vi "CPP-AQ.vi"() -> (5 "Plug in titles":string[](array[string]), 7 "Plug in values":string[](array[string]))   [LabVIEW 2016]
uses:
  <vilib>/Utility/miscctls.llb/LVPositionTypeDef.ctl
  <vilib>/Utility/miscctls.llb/LVForegroundBackgroundColorsTypeDef.ctl
  Globals/Meas_global.vi
  CPPSW/CPP Global.vi
panel:
  in  "Tab Control":enum32{"FID Traces", "Numerics"}(tab)
  out "FID Means":T1(graph)
  out "FID PPM":cluster{"Time (s)":dbl[], "Eng Values":dbl[]}[](graph)
  out "COV(%)":dbl[](array[numeric])
  out "sigma(ppm)":dbl[](array[numeric])
  out "DeltaMean(ppm)":dbl[](array[numeric])
  in  "Blocks":i32
  out "FIDsymbol":string[](array[string])
  out "PPM":dbl[](array[numeric]) format="%.1f"
  # "Avg PPM Above BG"
  # "https://en.wikipedia.org/wiki/Coefficient_of_variation"
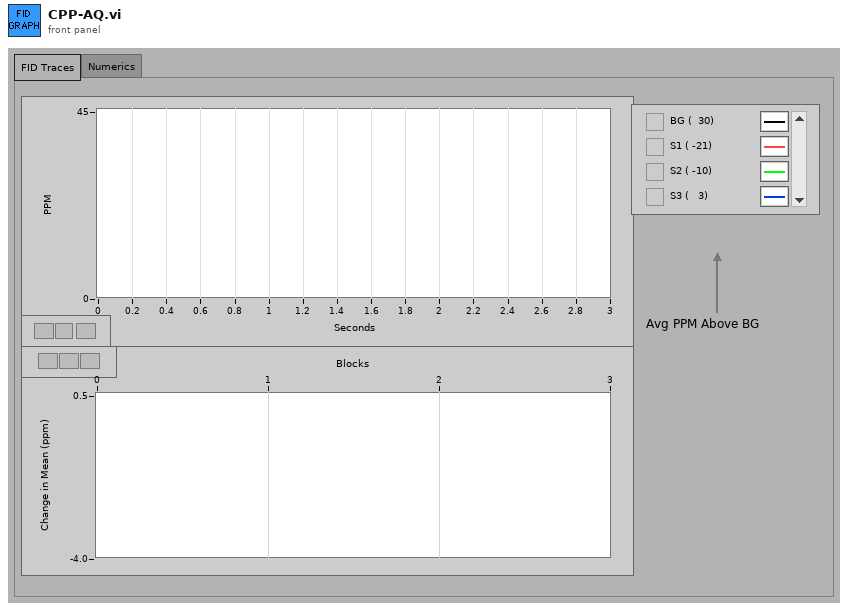
[diagram p1: front panel]
types:
  T1 = cluster{"[0]":dbl, "[1]":dbl, "[2]":dbl, "[3]":dbl}
  T2 = typedef "Analysis_info_cluster.ctl" = cluster{"Colour":u32, "Inst type":T3, "Inst name":string, "Symbol":string, "Code name":string, "Extra Info":string, "Inst Array":T4, "Extra Titles":string[], "Extra Values":string[], "U":dbl, "u^2":dbl, "u^3":dbl, "u^4":dbl, "Skew_u":dbl, "Kurt_u":dbl, "Sd Error in Mean":dbl, "% u'/U":dbl, "X":dbl, "Y":dbl, "Z":dbl, "Timescale integral Estimate":dbl, "Sd Error in Variance":dbl, "Calib File":path, "Calib Constants":dbl[], "Output Position":bool, "Full Stats":bool, "Av Sampling Rate":dbl, "Av No of Samples":dbl, "Total Meas Time (s)":dbl, "ADAM Ch Name":string, "Max value":dbl, "Min value":dbl}
  T3 = typedef "Inst_type.ctl" = enum16{"Propeller anemometer", "Raw voltage", "Pressure Transducer", "Pitot-static tube", "Preston tube", "Hot wire", "Cross wire 1", "Cross wire 2", "Generic Linear", "Generic Polynomial", "Generic BackPoly", "Fast FID", "Thermocouple", "Cold wire", "Pulsed Wire", "LDA Vel", "LDA Tran time", "LDA Arr time", "Microphone"}
  T4 = typedef "Instrument_Array.ctl" = enum16{"PWA", "LDA", "Analogue"}
  T5 = typedef "Time_Trace_Cluster.ctl" = cluster{"Weighting":dbl[], "Time (s)":dbl[], "Voltage":dbl[], "Eng Values":dbl[]}
  T6 = cluster{"[0]":dbl, "[1]":dbl, "[2]":dbl, "[3]":dbl}[]
  T7 = typedef "FIDmapping.ctl" = cluster{"Run #":dbl, "Run Suffix":u16, "Receptor #":u16, "ReceptorID":u16, "FIDname":string, "Long\nRun?":bool}[]
  T8 = cluster{"Receptor IDs":string[], "Receptor Numbers":u16[]}
  T9 = cluster{"Run #":dbl, "Run Suffix":u16, "Receptor #":u16, "ReceptorID":u16, "FIDname":string, "Long\nRun?":bool}
  T10 = typedef "LVPositionTypeDef.ctl" = cluster{"Left":i32, "Top":i32}
  T11 = typedef "LVForegroundBackgroundColorsTypeDef.ctl" = cluster{"Foreground Color":u32, "Background Color":u32}
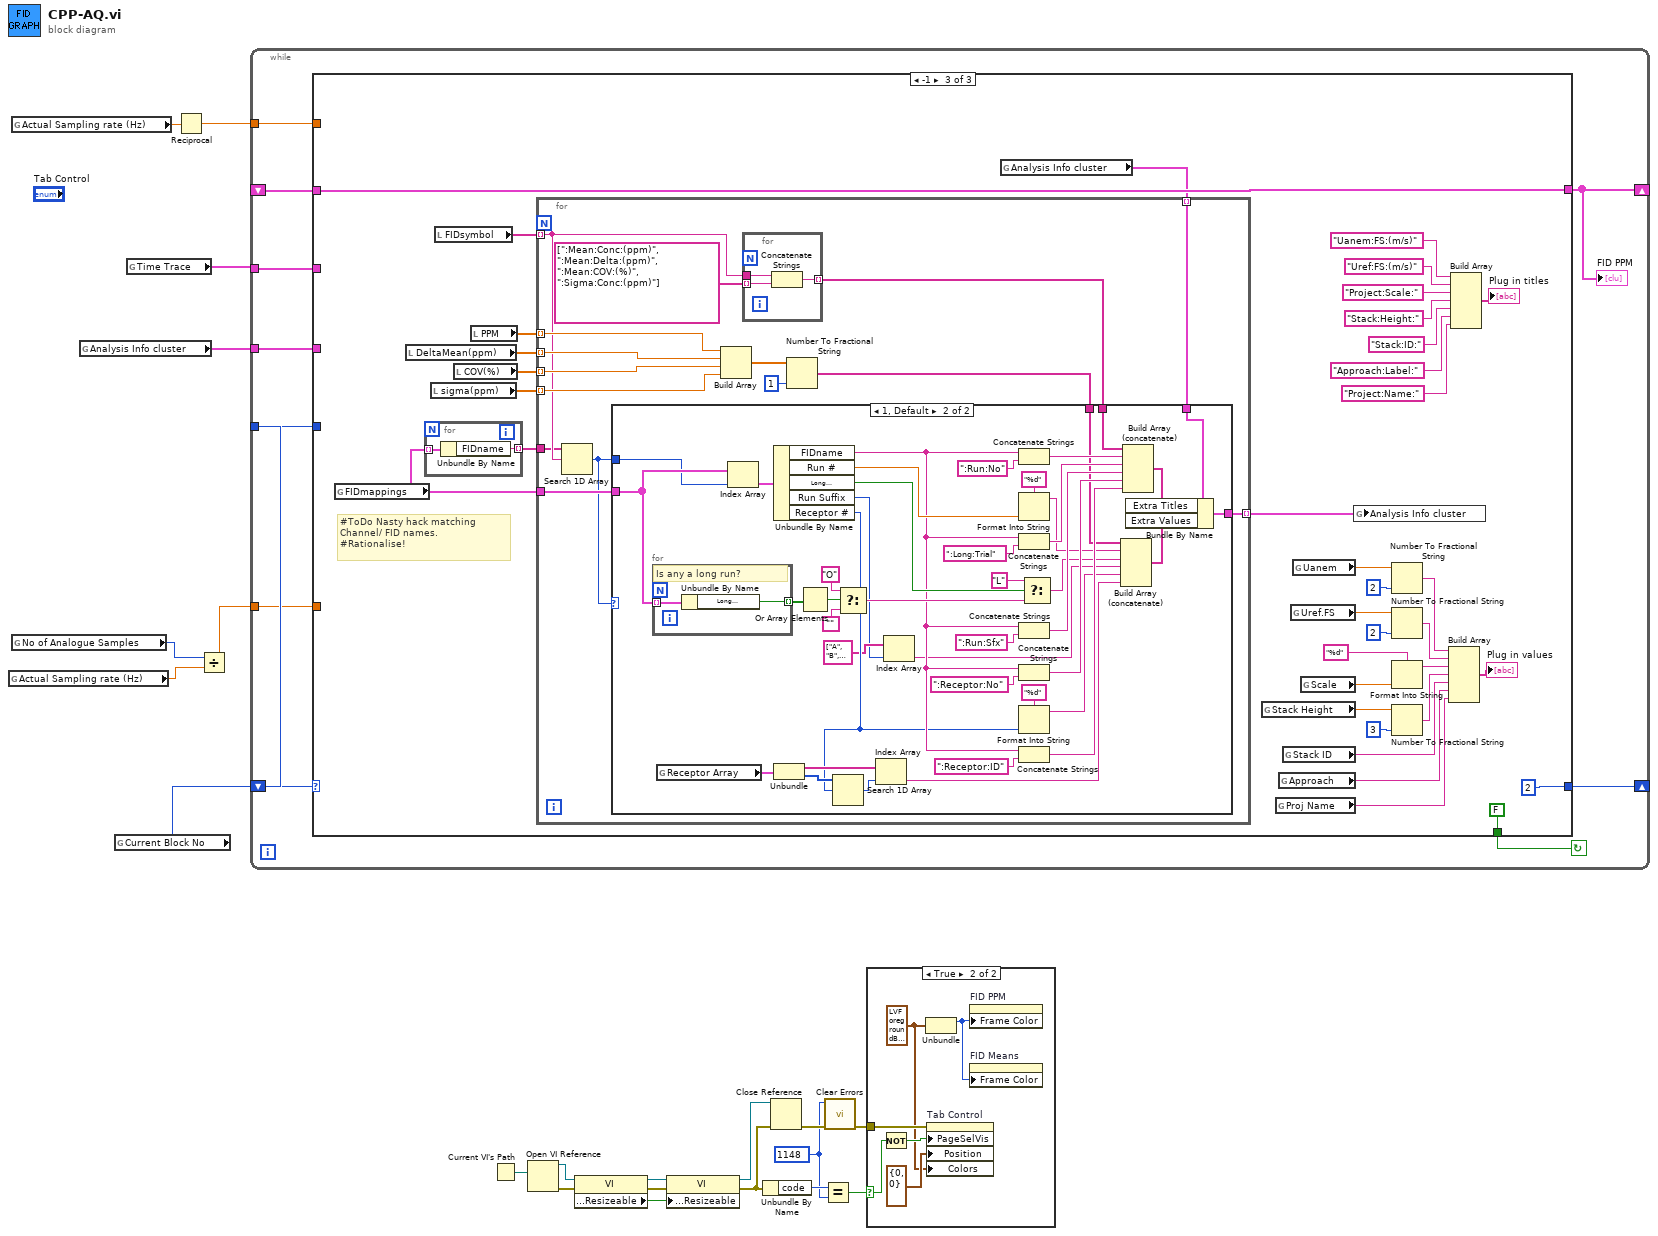
[diagram p0: block diagram]
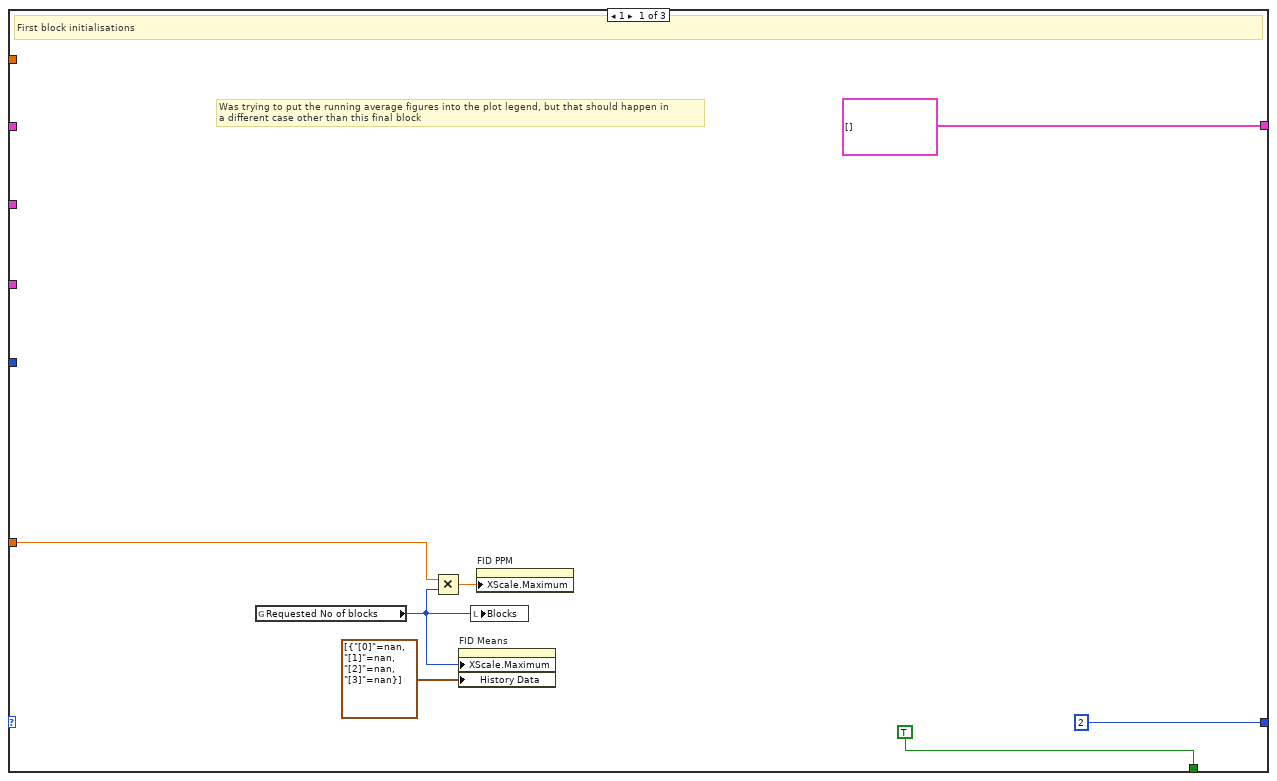
[diagram p3: hidden frame]
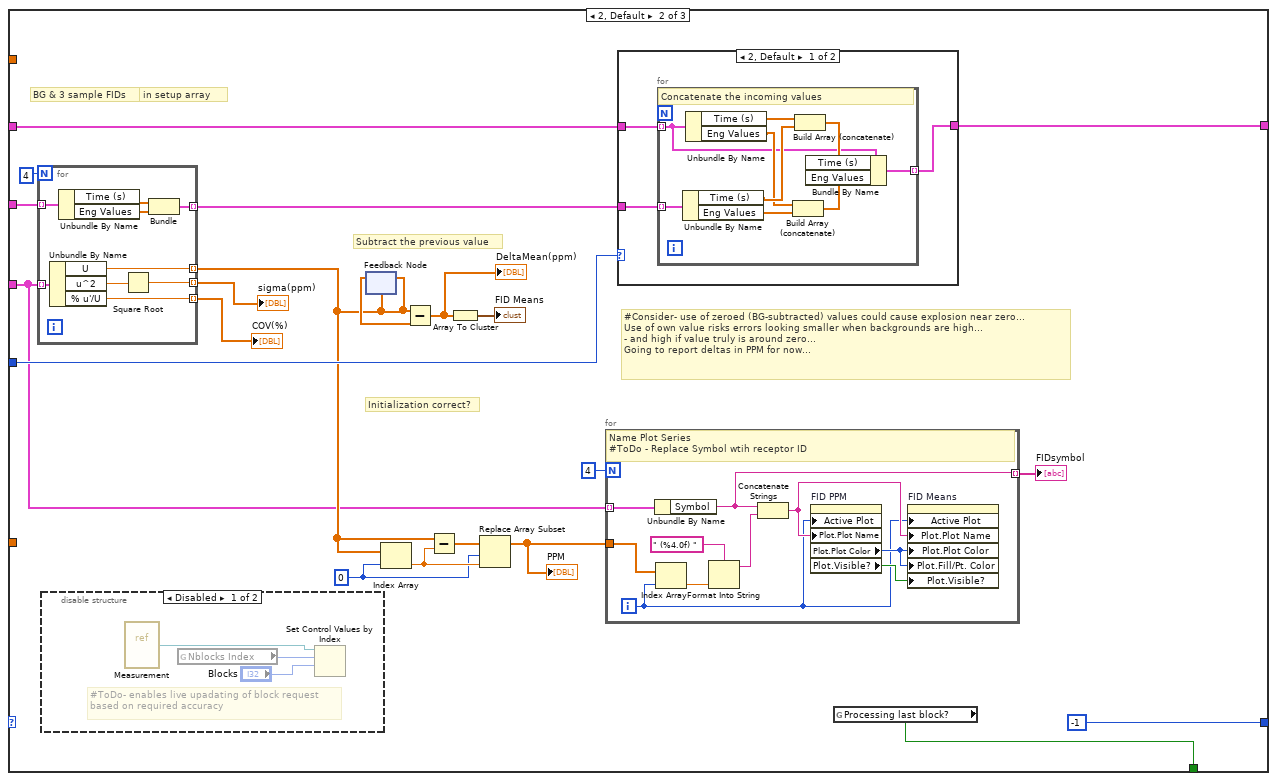
[diagram p4: hidden frame]
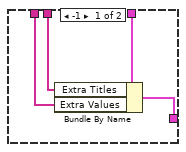
[diagram p7: hidden frame]
diagram:
  w3 = 1148 ("y")
  n1 = global read "Meas_global.vi" "Actual Sampling rate (Hz)"() -> (w17:dbl)
  n2 = global read "Meas_global.vi" "Actual Sampling rate (Hz)"() -> (w20:dbl)
  n3 = global read "Meas_global.vi" "No of Analogue Samples"() -> (w16:i32)
  n4 = global read "Meas_global.vi" "Analysis Info cluster"() -> (w14:T2[])
  n5 = global read "Meas_global.vi" "Current Block No"() -> (w18:i32)
  n6 = global read "Meas_global.vi" "Time Trace"() -> (w21:T5[])
  n7 = Reciprocal(x=w20) -> (1/x=w19:dbl)
  n8 = Divide(x=w16, y=w17) -> (x/y=w15:dbl)
  n9 = while {
    shift-left: w18 -> [w28]
    shift-right: [w29] -> _
    tunnel: w21 -> [w30]
    tunnel: w19 -> [w24]
    tunnel: w18 -> [w27]
    tunnel: w15 -> [w25]
    tunnel: w14 -> [w26]
    shift-right: [w22] -> _
    shift-left: _ -> [w23]
    stop <- w31 continue-if-true
    n10 = case shown="-1" w28 {
      tunnel: [TRUE w58 FALSE] -> w31
      tunnel: w30 -> [_ w59 _]
      tunnel: w24 -> [_ _ _]
      tunnel: [2 -1 ("Case") 2 ("Case")] -> w29
      tunnel: w27 -> [_ w51 _]
      tunnel: w25 -> [w35 _ _]
      tunnel: w26 -> [_ w39 _]
      tunnel: [cluster{"Time (s)":dbl[], "Eng Values":dbl[]}[] [] w52 w128] -> w22
      tunnel: w23 -> [_ w53 w128]
      frame 1 {
        # "Was trying to put the running average figures into the plot legend, but that should happen in\na different case other than this final block"
        # "First block initialisations"
        n11 = global read "Meas_global.vi" "Requested No of blocks"() -> (w32:i32)
        n12 = Multiply(x=w35, y=w32) -> (x*y=w36:dbl)
        n13 = property on="FID Means" class="WFChart (strict)"("XScale.Maximum"=w32, "History Data"=T6 [{"[0]"=nan, "[1]"=nan, "[2]"=nan, "[3]"=nan}]) -> ()  [unwired: 2 in, 2 out]
        n14 = local write "Blocks"(w32) -> ()
        n15 = property on="FID PPM" class="XYGraph (strict)"("XScale.Maximum"=w36) -> ()  [unwired: 2 in, 2 out]
      }
      frame 2, Default {
        w47 = 0 ("index")
        # "Initialization correct?"
        # "#Consider- use of zeroed (BG-subtracted) values could cause explosion near zero...\nUse of own value risks errors looking smaller when backgrounds are high...\n- and high if value truly is around zero...\nGoing to report deltas in PPM for now..."
        # "Subtract the previous value"
        # "BG FID is first element in setup array"
        # "BG & 3 sample FIDs"
        n16 = for {
          N: 4 -> [_]
          tunnel: w59 -> [w94] mode=indexing
          tunnel: w39 -> [w93] mode=indexing
          tunnel: [w92] -> w44 mode=indexing
          tunnel: [w89] -> w54 mode=indexing
          tunnel: [w87] -> w46 mode=indexing
          tunnel: [w86] -> w45 mode=indexing
          n17 = Unbundle By Name(w93) -> ("U"=w92:dbl, "u^2"=w88:dbl, "% u'/U"=w86:dbl)
          n18 = Unbundle By Name(w94) -> ("Time (s)"=w91:dbl[], "Eng Values"=w90:dbl[])
          n19 = Square Root(x=w88) -> (sqrt(x)=w87:dbl)
          n20 = Bundle("Time (s)"=w91, "Eng Values"=w90) -> (w89:cluster{"Time (s)":dbl[], "Eng Values":dbl[]})  [unwired: 1 in]
        }
        "sigma(ppm)" <- w46
        "COV(%)" <- w45
        n21 = disable-structure shown="Disabled" {
          frame Disabled {
            # "#ToDo- enables live upadating of block request based on required accuracy"
            n22 = vi-ref "Measurement.vi"() -> (w61:refnum<vi>)
            n23 = global read "Meas_global.vi" "Nblocks Index"() -> (w62:i32)
            n24 = Set Control Values by Index(0:w61, 1:w62, 2:"Blocks") -> ()  [unwired: 1 in, 1 out]
          }
          frame Enabled {
          }
        }
        n25 = feedback-in #1(w44) -> ()
        n26 = feedback #1(w44) -> (w55:dbl[])
        n27 = Index Array(array=w44, index=w47) -> (element=w48:dbl)
        n28 = Subtract(x=w44, y=w55) -> (x-y=w43:dbl[])
        "DeltaMean(ppm)" <- w43
        n29 = Subtract(x=w44, y=w48) -> (x-y=w49:dbl[])
        n30 = Array To Cluster(array=w43) -> (cluster=→"FID Means":T1)
        n31 = Replace Array Subset(array=w49, new element=w48, index=w47) -> (w40:dbl[])
        "PPM" <- w40
        n32 = for {
          N: 4 -> [_]
          tunnel: w39 -> [w72] mode=indexing
          tunnel: [w63] -> w41 mode=indexing
          tunnel: w40 -> [w66]
          i -> [w65]
          # "Name Plot Series\n#ToDo - Replace Symbol wtih receptor ID"
          n33 = Unbundle By Name(w72) -> ("Symbol"=w63:string)
          n34 = Index Array(array=w66, index=w65) -> (element=w64:dbl)
          n35 = Format Into String(format string=" (%4.0f) ", w64) -> (resulting string=w67:string)  [unwired: 2 in, 1 out]
          n36 = Concatenate Strings(w63, w67) -> (w69:string)
          n37 = property on="FID PPM" class="XYGraph (strict)"("Active Plot"=w65, "Plot.Plot Name"=w69) -> ("Plot.Plot Color"=w71:u32, "Plot.Visible?"=w70:bool)  [unwired: 2 in, 2 out]
          n38 = property on="FID Means" class="WFChart (strict)"("Active Plot"=w65, "Plot.Plot Name"=w69, "Plot.Plot Color"=w71, "Plot.Fill/Pt. Color"=w71, "Plot.Visible?"=w70) -> ()  [unwired: 2 in, 2 out]
        }
        "FIDsymbol" <- w41
        n39 = case shown="2, Default" w51 {
          tunnel: [w73 w85] -> w52
          tunnel: w54 -> [w75 w85]
          tunnel: w53 -> [w74 _]
          frame 2, Default {
            n40 = for {
              tunnel: w74 -> [w77] mode=indexing
              tunnel: w75 -> [w76] mode=indexing
              tunnel: [w78] -> w73 mode=indexing
              # "Concatenate the incoming values"
              n41 = Unbundle By Name(w76) -> ("Time (s)"=w83:dbl[], "Eng Values"=w82:dbl[])
              n42 = Unbundle By Name(w77) -> ("Time (s)"=w84:dbl[], "Eng Values"=w81:dbl[])
              n43 = Build Array (concatenate)(w81, w82) -> (w79:dbl[])
              n44 = Build Array (concatenate)(w84, w83) -> (w80:dbl[])
              n45 = Bundle By Name(cluster=w77, "Time (s)"=w80, "Eng Values"=w79) -> (w78:cluster{"Time (s)":dbl[], "Eng Values":dbl[]})
            }
          }
          frame 1 {
            # "Initialise with first block of data"
          }
        }
        n46 = global read "Meas_global.vi" "Processing last block?"() -> (w58:bool)
      }
      frame -1 {
        # "#ToDo Nasty hack matching Channel/ FID names.\n#Rationalise!"
        n47 = global read "CPP Global.vi" "FIDmappings"() -> (w120:T7)
        n48 = local read "DeltaMean(ppm)"() -> (w122:dbl[])
        n49 = for {
          tunnel: w120 -> [w132] mode=indexing
          tunnel: [w131] -> w119 mode=indexing
          n50 = Unbundle By Name(w132) -> ("FIDname"=w131:string)
        }
        n51 = local read "sigma(ppm)"() -> (w123:dbl[])
        n52 = local read "FIDsymbol"() -> (w127:string[])
        n53 = local read "COV(%)"() -> (w121:dbl[])
        n54 = local read "PPM"() -> (w124:dbl[])
        n55 = global read "Meas_global.vi" "Analysis Info cluster"() -> (w126:T2[])
        n56 = for {
          tunnel: w127 -> [w135] mode=indexing
          tunnel: w126 -> [w144] mode=indexing
          tunnel: [w143] -> w125 mode=indexing
          tunnel: w124 -> [w142] mode=indexing
          tunnel: w123 -> [w141] mode=indexing
          tunnel: w122 -> [w140] mode=indexing
          tunnel: w121 -> [w139] mode=indexing
          tunnel: w120 -> [w138]
          tunnel: w119 -> [w134]
          n57 = Search 1D Array(1D array=w134, element=w135) -> (index of element=w133:i32)  [unwired: 1 in]
          n58 = Build Array(w142, w140, w139, w141) -> (w147:dbl[])
          n59 = for {
            tunnel: w135 -> [w198]
            tunnel: string[] [":Mean:Conc:(ppm)", ":Mean:Delta:(ppm)", ":Mean:COV:(%)", ":Sigma:Conc:(ppm)"] -> [w197] mode=indexing
            tunnel: [w196] -> w137 mode=indexing
            n60 = Concatenate Strings(w198, w197) -> (w196:string)
          }
          n61 = Number To Fractional String(number=w147, precision (6)=i16 1) -> (F-format string=w136:string[])  [unwired: 2 in]
          n62 = case shown="1, Default" w133 {
            tunnel: w144 -> [w151 w193]
            tunnel: [w150 w192] -> w143
            tunnel: w138 -> [_ w170]
            tunnel: w137 -> [w149 w164]
            tunnel: w136 -> [w148 w159]
            tunnel: w133 -> [_ w155]
            frame -1 {
              n63 = Bundle By Name(cluster=w151, "Extra Titles"=w149, "Extra Values"=w148) -> (w150:T2)
            }
            frame 1, Default {
              n64 = for {
                tunnel: w170 -> [w195] mode=indexing
                tunnel: [w194] -> w191 mode=indexing
                # "Is any a long run?"
                n65 = Unbundle By Name(w195) -> ("Long\nRun?"=w194:bool)
              }
              n66 = global read "CPP Global.vi" "Receptor Array"() -> (w174:T8)
              n67 = Index Array(array=w170, index=w155) -> (element=w171:T9)
              n68 = Unbundle By Name(w171) -> ("FIDname"=w176:string, "Run #"=w185:dbl, "Long\nRun?"=w183:bool, "Run Suffix"=w153:u16, "Receptor #"=w156:u16)
              n69 = Unbundle(w174) -> ("Receptor IDs"=w172:string[], "Receptor Numbers"=w173:u16[])
              n70 = Or Array Elements(Boolean array=w191) -> (logical OR=w190:bool)
              n71 = Search 1D Array(1D array=w173, element=w156) -> (index of element=w175:i32)  [unwired: 1 in]
              n72 = Select(t="O" ("string"), s=w190, f="") -> (s? t:f=w187:string)
              n73 = Index Array(array=w172, index=w175) -> (element=w160:string)
              n74 = Index Array(array=string[] ["A", "B", "C", "D", "E", "F", "G", "H", "I", "J", "K", "L", "M", "N", "O", "P", "Q", "R", "S", "T", "U", "V", "W", "X", "Y", "Z"], index=w153) -> (element=w152:string)
              n75 = Concatenate Strings(w176, ":Run:No" ("string")) -> (w169:string)
              n76 = Format Into String(format string="%d", w185) -> (resulting string=w163:string)  [unwired: 2 in, 1 out]
              n77 = Concatenate Strings(w176, ":Long:Trial" ("string")) -> (w168:string)
              n78 = Concatenate Strings(w176, ":Run:Sfx" ("string")) -> (w167:string)
              n79 = Concatenate Strings(w176, ":Receptor:No" ("string")) -> (w166:string)
              n80 = Format Into String(format string="%d", w156) -> (resulting string=w161:string)  [unwired: 2 in, 1 out]
              n81 = Concatenate Strings(w176, ":Receptor:ID" ("string")) -> (w165:string)
              n82 = Select(t="L" ("string"), s=w183, f=w187) -> (s? t:f=w162:string)
              n83 = Build Array (concatenate)(w159, w163, w162, w152, w161, w160) -> (w157:string[])
              n84 = Build Array (concatenate)(w164, w169, w168, w167, w166, w165) -> (w158:string[])
              n85 = Bundle By Name(cluster=w193, "Extra Titles"=w158, "Extra Values"=w157) -> (w192:T2)
            }
          }
        }
        n86 = global read "CPP Global.vi" "Stack Height"() -> (w103:dbl)
        n87 = global read "CPP Global.vi" "Proj Name"() -> (w96:string)
        n88 = global read "CPP Global.vi" "Approach"() -> (w100:string)
        n89 = global read "CPP Global.vi" "Stack ID"() -> (w101:string)
        n90 = global read "CPP Global.vi" "Uref.FS"() -> (w98:dbl)
        n91 = global read "CPP Global.vi" "Uanem"() -> (w110:dbl)
        n92 = global read "CPP Global.vi" "Scale"() -> (w106:dbl)
        n93 = global write "Meas_global.vi" "Analysis Info cluster"(w125) -> ()
        n94 = Number To Fractional String(number=w110, precision (6)=i16 2) -> (F-format string=w108:string)  [unwired: 2 in]
        n95 = Number To Fractional String(number=w98, precision (6)=i16 2) -> (F-format string=w97:string)  [unwired: 2 in]
        n96 = Format Into String(format string="%d", w106) -> (resulting string=w105:string)  [unwired: 2 in, 1 out]
        n97 = Number To Fractional String(number=w103, precision (6)=i16 3) -> (F-format string=w102:string)  [unwired: 2 in]
        n98 = Build Array(w108, w97, w105, w102, w101, w100, w96) -> (→"Plug in values":string[])
        n99 = Build Array("Uanem:FS:(m/s)", "Uref:FS:(m/s)" ("element"), "Project:Scale:", "Stack:Height:", "Stack:ID:", "Approach:Label:", "Project:Name:") -> (→"Plug in titles":string[])
      }
    }
    "FID PPM" <- w22
  }
  n100 = Current VI's Path() -> (path=w6:path)
  n101 = Open VI Reference(vi path=w6) -> (vi reference=w7:refnum<vi>, error out=w8:errorcluster)  [unwired: 5 in]
  n102 = property class="VI"(reference=w7, error in=w8) -> (reference out=w9:refnum<vi>, error out=w10:errorcluster, "Front Panel.Resizeable"=w11:bool)
  n103 = property class="VI"(reference=w9, error in=w10, "Front Panel.Resizeable"=w11) -> (reference out=w12:refnum<vi>, error out=w5:errorcluster)
  n104 = Unbundle By Name(w5) -> ("code"=w13:i32)
  n105 = Close Reference(reference=w12, error in (no error)=w5) -> (error out=w4:errorcluster)
  n106 = Equal?(x=w13, y=w3) -> (x = y?=w1:bool)
  n107 = call <vilib>:"Clear Errors.vi"("error in (no error)"=w4, "specific error code to clear (0: all)"=w3) -> ("error out"=w2:errorcluster)  [unwired: 4 in, 1 out]
  n108 = case shown="True" w1 {
    selector: w1 -> [_ w201]
    tunnel: w2 -> [_ w204]
    frame False {
    }
    frame True {
      w200 = T11 {"Foreground Color"=16750848, "Background Color"=16750848} ("Colors")
      n109 = Not(x=w201) -> (.not. x?=w203:bool)
      n110 = Unbundle(w200) -> ("Foreground Color"=w199:u32)  [unwired: 1 out]
      n111 = property on="Tab Control" class="TabCtl (strict)"(error in=w204, "PageSelVis"=w203, "Position"=T10 {"Left"=0, "Top"=0}, "Colors"=w200) -> ()  [unwired: 1 in, 2 out]
      n112 = property on="FID PPM" class="XYGraph (strict)"("Frame Color"=w199) -> ()  [unwired: 2 in, 2 out]
      n113 = property on="FID Means" class="WFChart (strict)"("Frame Color"=w199) -> ()  [unwired: 2 in, 2 out]
    }
  }
